vi "List Feeds and Packages in the SystemLink Repository.vi"() -> ()   [LabVIEW 2025]
doc: "This example shows how to open a connection to the SystemLink server and get a list of the feeds and packages in the SystemLink server's repository."
uses:
  Open SystemLink Connection (Basic).vi
  Open SystemLink Connection (API Key).vi
  SystemLink_Repo_API.lvlib
panel:
  in  "Login Options":enum32{"Username and Password", "API Key"}(tab)
  in  "Username":string
  in  "Password":string
  in  "API Key":string
  in  "SystemLink server base URL":string="https://"
  out "List of all Packages in the SystemLink Repository":string[][](table)
  out "List of Feeds in the SystemLink Repository":string[](array[string])
  # "SystemLink Server"
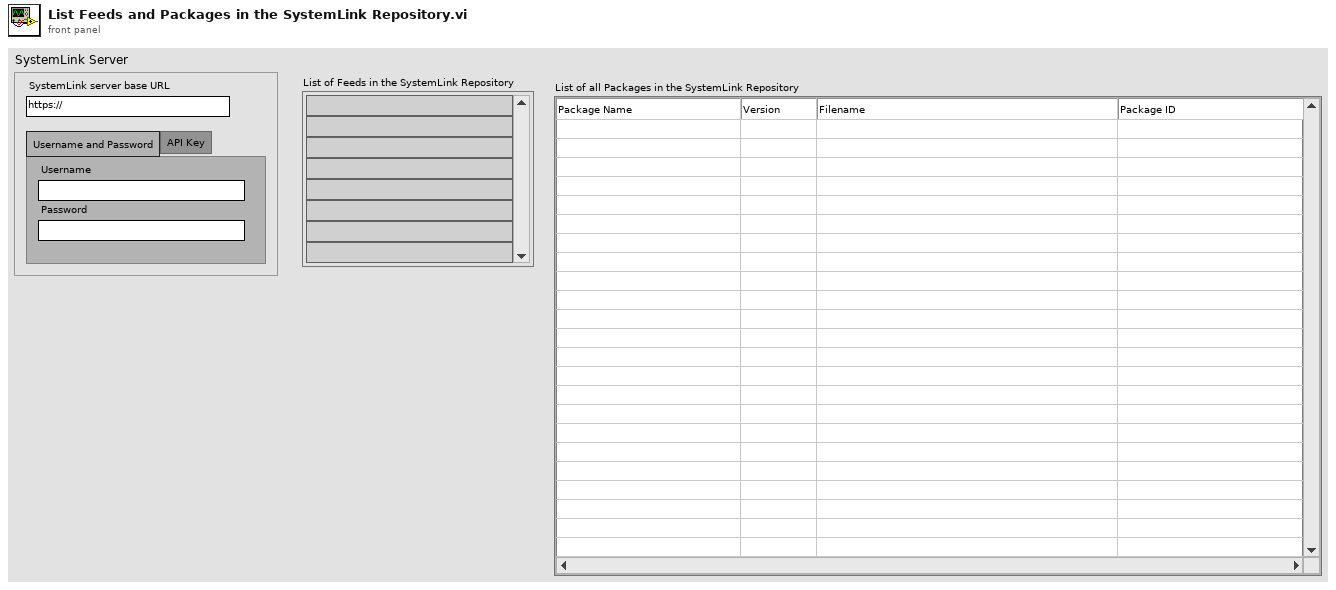
[diagram p1: front panel]
types:
  T1 = typedef "SystemLink_Repo_API.lvlib/systemlink repo.ctl" = cluster{"client handle out":T2, "SystemLink server base URL":string}
  T2 = typedef "LabVIEWHTTPClient.lvlib/ClientHandle.ctl" = refnum<k1>
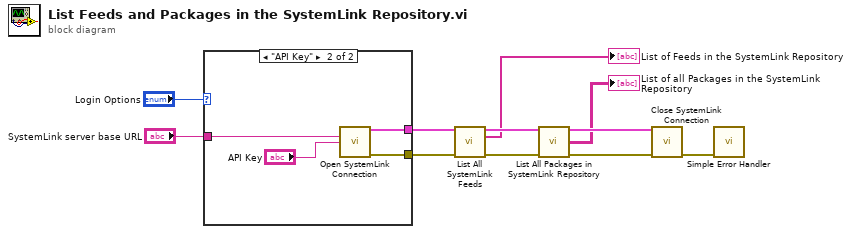
[diagram p0: block diagram]
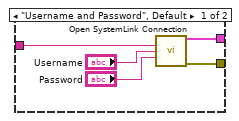
[diagram p2: hidden frame]
diagram:
  n1 = case shown="\"API Key\"" "Login Options" {
    tunnel: [w16 w20] -> w1
    tunnel: [w15 w19] -> w2
    tunnel: "SystemLink server base URL" -> [w12 w18]
    frame "Username and Password", Default {
      n2 = call-poly "Open SystemLink Connection.vi"("SystemLink server base URL"=w12, "username"="Username", "password"="Password") -> ("SystemLink repo out"=w16:T1, "error out"=w15:errorcluster)  [unwired: 11 in]
    }
    frame "API Key" {
      n3 = call-poly "Open SystemLink Connection.vi"("SystemLink server base URL"=w18, "API Key"="API Key") -> ("SystemLink repo out"=w20:T1, "error out"=w19:errorcluster)  [unwired: 12 in]
    }
  }
  n4 = call "List All SystemLink Feeds.vi"("SystemLink repo in"=w1, "error in (no error)"=w2) -> ("SystemLink repo out"=w11:T1, "SystemLink Feed Names"=→"List of Feeds in the SystemLink Repository":string[], "error out"=w9:errorcluster)  [unwired: 10 in, 1 out]
  n5 = call "List All Packages in SystemLink Repository.vi"("SystemLink repo in"=w11, "error in (no error)"=w9) -> ("SystemLink repo out"=w10:T1, "packages"=→"List of all Packages in the SystemLink Repository":string[][], "error out"=w8:errorcluster)  [unwired: 11 in]
  n6 = call "Close SystemLink Connection.vi"("SystemLink repo in"=w10, "error in (no error)"=w8) -> ("error out"=w5:errorcluster)  [unwired: 13 in]
  n7 = call <vilib>:"Simple Error Handler.vi"("error in (no error)"=w5) -> ()  [unwired: 4 in, 5 out]
